vi "Load Signal Bank.vi"(5 "Input array":dbl[][](array[numeric])=array10000x1[10000 elements] format="%.2f", 6 "CCA":cluster{"channel":string, "channel on":bool}[](array[cluster])=[{"channel"="0", "channel on"=TRUE}, {"channel"="1", "channel on"=TRUE}, {"channel"="2", "channel on"=TRUE}, {"channel"="3", "channel on"=TRUE}, {"channel"="4", "channel on"=FALSE}, {"channel"="5", "channel on"=FALSE}, {"channel"="6", "channel on"=FALSE}, {"channel"="7", "channel on"=FALSE}]) -> ()   [LabVIEW 2015]
uses:
  DAQ Engine VIs/PXI Globals.vi
panel:
  in  "Action":enum16{"Add", "Replace ID", "Read ID", "Clear"}(ring)
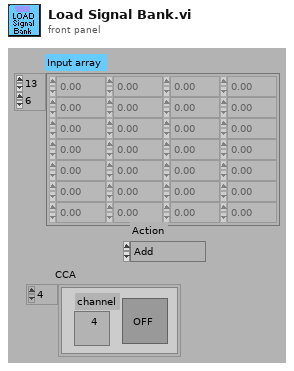
[diagram p1: front panel]
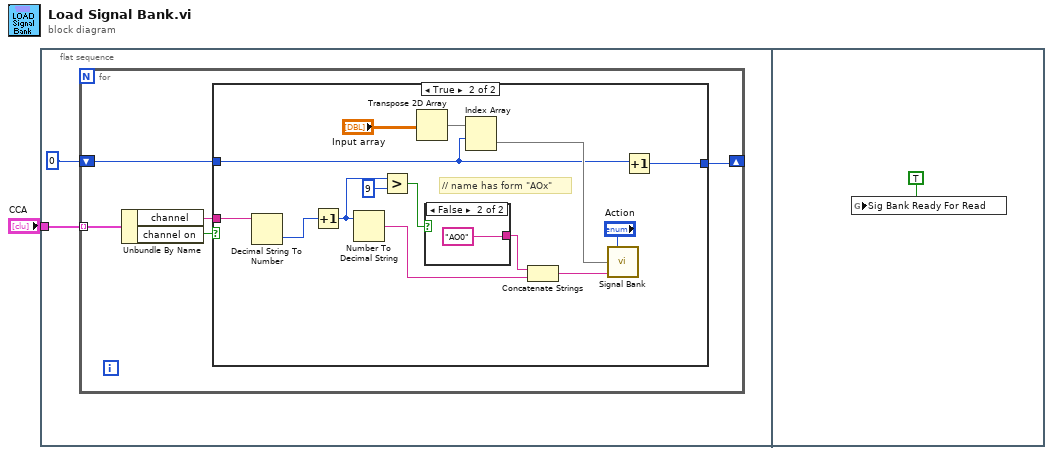
[diagram p0: block diagram]
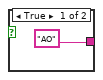
[diagram p3: hidden frame]
diagram:
  n1 = flat-sequence {
    tunnel: "CCA" -> [w2]
    frame #0 {
      n2 = for {
        tunnel: w2 -> [w8] mode=indexing
        shift-right: [w4] -> _
        shift-left: 0 -> [w5]
        n3 = Unbundle By Name(w8) -> ("channel"=w7:string, "channel on"=w6:bool)
        n4 = case shown="True" w6 {
          tunnel: w7 -> [_ w15]
          tunnel: w5 -> [w9 w18]
          tunnel: [w9 w19] -> w4
          frame False {
          }
          frame True {
            # "// name has form \"AOx\""
            n5 = Decimal String To Number(string=w15) -> (number=w14:i32)  [unwired: 2 in, 1 out]
            n6 = Increment(x=w14) -> (x+1=w11:i32)
            n7 = Number To Decimal String(number=w11) -> (decimal integer string=w16:string)  [unwired: 1 in]
            n8 = Greater?(x=w11, y=9) -> (0:w12:bool)
            n9 = Transpose 2D Array(2D array="Input array") -> (transposed array=w17:dbl[][])
            n10 = case shown="False" w12 {
              tunnel: ["AO" "AO0"] -> w10
              frame True {
              }
              frame False {
              }
            }
            n11 = Index Array(array=w17, index (row)=w18) -> (element=w20:dbl[])  [unwired: 1 in]
            n12 = Concatenate Strings(w10, w16) -> (w23:string)
            n13 = call "Signal Bank.vi"("Action"="Action", "1D Data In"=w20, "ID"=w23) -> ()  [unwired: 11 in, 2 out]
            n14 = Increment(x=w18) -> (x+1=w19:i32)
          }
        }
      }
    }
    frame #1 {
      n15 = global write "PXI Globals.vi" "Sig Bank Ready For Read"(TRUE) -> ()
    }
  }
